vi "Data Read Multi Points.vi"(0 "VISA resource name":refnum<visa-resource-name>, 2 "Sample Count (1)":i32=1 min=1 max=50000, 3 "Timeout (10000 ms)":i32=10000 format="%#.6g", 5 "error in (no error)":errorcluster) -> (14 "VISA resource name out":refnum<visa-resource-name>, 16 "Measurements":dbl[](array[numeric]), 19 "error out":errorcluster)   [LabVIEW 2020, in "Keithley 2100 Series.lvlib"]
doc: "Reads and returns multiple measurements from the instrument. Use this VI when you want to take multiple measurements using an immediate trigger. Use the low-level VIs for other triggering options."
uses:
  Keithley 2100 Series.lvlib
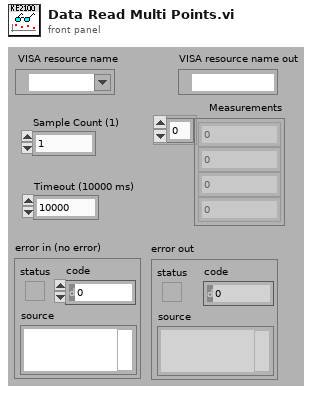
[diagram p1: front panel]
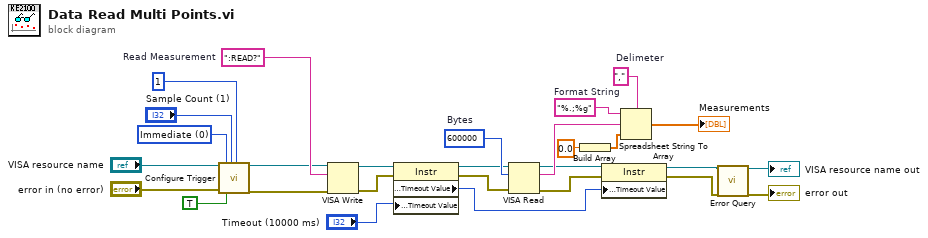
[diagram p0: block diagram]
diagram:
  w2 = u16 0 items=["Immediate", "Bus", "External"] ("Source (0: Immediate)")
  w23 = ","  # Delimeter
  w24 = "%.;%g"  # Format String
  w14 = ":READ?"  # Read Measurement
  w26 = u32 600000  # Bytes
  n1 = call "Configure Trigger.vi"("VISA resource name"="VISA resource name", "error in (no error)"="error in (no error)", "Source (0: Immediate)"=w2, "Auto Delay? (T: Auto)"=TRUE, "Sample Count (1)"="Sample Count (1)", "Trigger Count (1)"=1) -> ("VISA resource name out"=w5:refnum<visa-resource-name>, "error out"=w6:errorcluster)  [unwired: 12 in]
  n2 = VISA Write(VISA resource name=w5, write buffer=w14, error in (no error)=w6) -> (VISA resource name out=w13:refnum<visa-resource-name>, error out=w12:errorcluster)  [unwired: 1 out]
  n3 = property class="Instr"(reference=w13, error in=w12, "General Settings:Timeout Value"="Timeout (10000 ms)") -> (reference out=w20:refnum<visa-resource-name>, error out=w19:errorcluster, "General Settings:Timeout Value"=w15:u32)
  n4 = VISA Read(VISA resource name=w20, byte count=w26, error in (no error)=w19) -> (VISA resource name out=w17:refnum<visa-resource-name>, read buffer=w25:string, error out=w16:errorcluster)  [unwired: 1 out]
  n5 = Build Array(0.0) -> (w21:dbl[])
  n6 = property class="Instr"(reference=w17, error in=w16, "General Settings:Timeout Value"=w15) -> (reference out=w11:refnum<visa-resource-name>, error out=w10:errorcluster)
  n7 = Spreadsheet String To Array(delimiter (Tab)=w23, format string=w24, spreadsheet string=w25, array type (2D Dbl)=w21) -> (array=→"Measurements":dbl[])
  n8 = call "Error Query.vi"("VISA resource name"=w11, "error in (no error)"=w10) -> ("VISA resource name out"=→"VISA resource name out":refnum<visa-resource-name>, "error out"=→"error out":errorcluster)  [unwired: 14 in, 2 out]
